vi "Benchmark.vi"() -> ()   [LabVIEW 2023]
uses:
  <vilib>/vision/NI_Vision_Development_Module.lvlib
  WrapperSubVIs/Wrapper.dll
panel:
  out "Time per Image, µs ipp":dbl
  out "Time per Image, µs NI 2 no try catch":dbl
  out "Time per Image, µs 3":dbl
  out "Time per Image, µs 2":dbl
  out "Time per Image, µs original NI":dbl
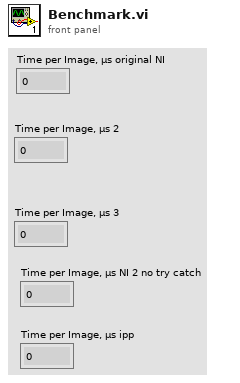
[diagram p1: front panel]
types:
  T1 = typedef "Image Type" = u32
  T2 = typedef "IMAQ Image.ctl" = refnum<image>
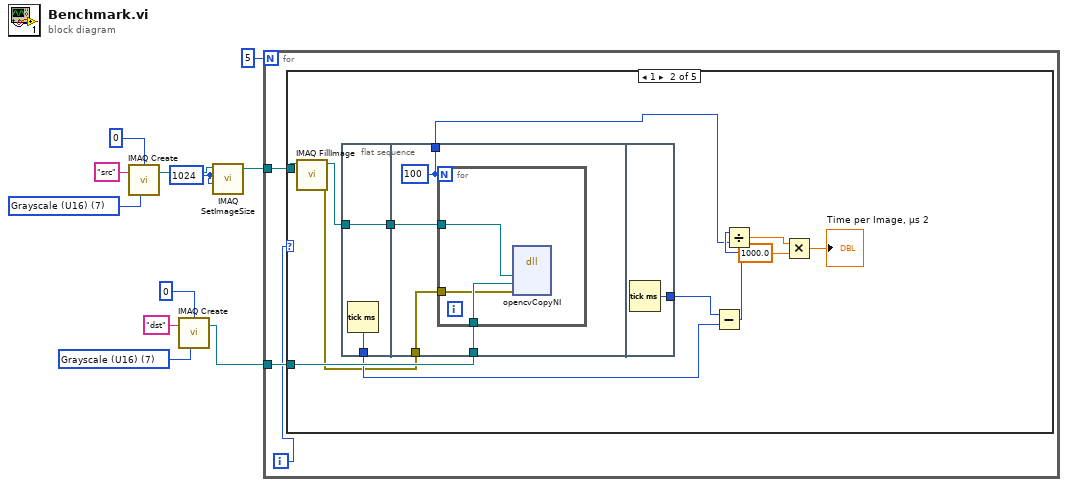
[diagram p0: block diagram]
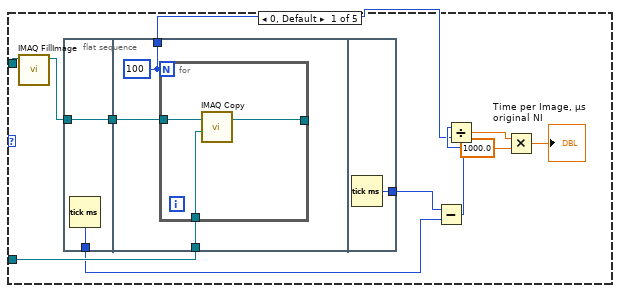
[diagram p2: hidden frame]
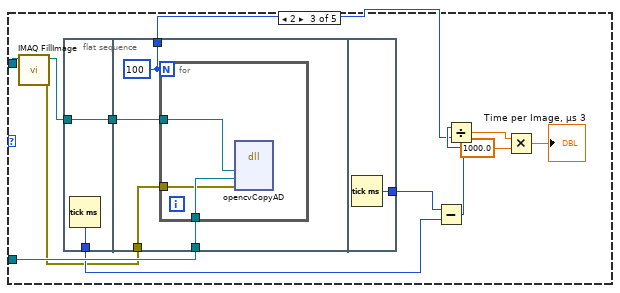
[diagram p3: hidden frame]
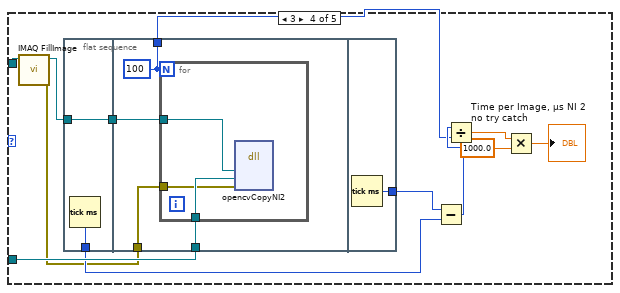
[diagram p4: hidden frame]
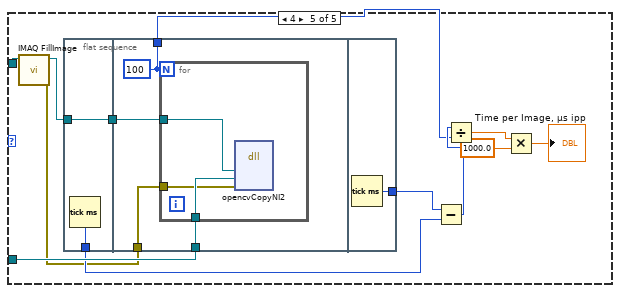
[diagram p5: hidden frame]
diagram:
  w5 = T1 7 items=["Grayscale (U8)", "Grayscale (I16)", "Grayscale (SGL)", "Complex (CSG)", "RGB (U32)", "HSL (U32)", "RGB (U64)", "Grayscale (U16)"] ("Image Type")
  w8 = 1024 ("X Resolution")
  w10 = T1 7 items=["Grayscale (U8)", "Grayscale (I16)", "Grayscale (SGL)", "Complex (CSG)", "RGB (U32)", "HSL (U32)", "RGB (U64)", "Grayscale (U16)"] ("Image Type")
  n1 = call "IMAQ Create"("Border Size"=0, "Image Name"="src", "Image Type"=w10) -> ("New Image"=w9:T2)  [unwired: 2 in, 1 out]
  n2 = call "IMAQ Create"("Border Size"=0, "Image Name"="dst", "Image Type"=w5) -> ("New Image"=w2:T2)  [unwired: 2 in, 1 out]
  n3 = call "IMAQ SetImageSize"("Y Resolution"=w8, "X Resolution"=w8, "Image"=w9) -> ("Image Out"=w3:T2)  [unwired: 2 in, 1 out]
  n4 = for {
    N: 5 -> [_]
    tunnel: w3 -> [w14]
    tunnel: w2 -> [w13]
    i -> [w12]
    n5 = case shown="1" w12 {
      tunnel: w14 -> [w24 w45 w67 w89 w111]
      tunnel: w13 -> [w22 w43 w65 w87 w109]
      frame 0, Default {
        n6 = call "IMAQ FillImage"("Image"=w24) -> ("Image Out"=w23:T2)  [unwired: 9 in, 1 out]
        n7 = flat-sequence {
          tunnel: w23 -> [w27]
          tunnel: [w27] -> w25
          tunnel: [w26] -> w20
          tunnel: w25 -> [w30]
          tunnel: w22 -> [w29]
          tunnel: [w28] -> w18
          tunnel: [w34] -> w21
          frame #0 {
            n8 = Tick Count (ms)() -> (millisecond timer value=w26:u32)
          }
          frame #1 {
            w28 = 100
            n9 = for {
              N: w28 -> [_]
              tunnel: w30 -> [w33]
              tunnel: w29 -> [w32]
              tunnel: [w31] -> _
              n10 = call "IMAQ Copy"("Image Dst"=w32, "Image Src"=w33) -> ("Image Dst Out"=w31:T2)  [unwired: 4 in, 1 out]
            }
          }
          frame #2 {
            n11 = Tick Count (ms)() -> (millisecond timer value=w34:u32)
          }
        }
        n12 = Subtract(x=w21, y=w20) -> (x-y=w19:u32)
        n13 = Divide(x=w19, y=w18) -> (x/y=w17:dbl)
        n14 = Multiply(x=w17, y=1000.0) -> (x*y=→"Time per Image, µs original NI":dbl)
      }
      frame 1 {
        n15 = call "IMAQ FillImage"("Image"=w45) -> ("error out"=w35:errorcluster, "Image Out"=w44:T2)  [unwired: 9 in]
        n16 = flat-sequence {
          tunnel: w44 -> [w48]
          tunnel: [w48] -> w46
          tunnel: [w47] -> w41
          tunnel: w46 -> [w52]
          tunnel: w43 -> [w51]
          tunnel: [w50] -> w39
          tunnel: w35 -> [w49]
          tunnel: [w56] -> w42
          frame #0 {
            n17 = Tick Count (ms)() -> (millisecond timer value=w47:u32)
          }
          frame #1 {
            w50 = 100
            n18 = for {
              N: w50 -> [_]
              tunnel: w52 -> [w55]
              tunnel: w51 -> [w54]
              tunnel: w49 -> [w53]
              n19 = dll-call lib="C:/Users/Andrey/Desktop/xe2/WrapperSubVIs/Wrapper.dll" fn="opencvCopyNI"("src"=w55, "dst"=w54, "err"=w53) -> ()  [unwired: 7 in, 2 out]
            }
          }
          frame #2 {
            n20 = Tick Count (ms)() -> (millisecond timer value=w56:u32)
          }
        }
        n21 = Subtract(x=w42, y=w41) -> (x-y=w40:u32)
        n22 = Divide(x=w40, y=w39) -> (x/y=w38:dbl)
        n23 = Multiply(x=w38, y=1000.0) -> (x*y=→"Time per Image, µs 2":dbl)
      }
      frame 2 {
        n24 = call "IMAQ FillImage"("Image"=w67) -> ("error out"=w57:errorcluster, "Image Out"=w66:T2)  [unwired: 9 in]
        n25 = flat-sequence {
          tunnel: w66 -> [w70]
          tunnel: [w70] -> w68
          tunnel: [w69] -> w63
          tunnel: w68 -> [w74]
          tunnel: w65 -> [w73]
          tunnel: [w72] -> w61
          tunnel: w57 -> [w71]
          tunnel: [w78] -> w64
          frame #0 {
            n26 = Tick Count (ms)() -> (millisecond timer value=w69:u32)
          }
          frame #1 {
            w72 = 100
            n27 = for {
              N: w72 -> [_]
              tunnel: w74 -> [w77]
              tunnel: w73 -> [w76]
              tunnel: w71 -> [w75]
              n28 = dll-call lib="C:/Users/Andrey/Desktop/xe2/WrapperSubVIs/Wrapper.dll" fn="opencvCopyAD"("src"=w77, "dst"=w76, "err"=w75) -> ()  [unwired: 7 in, 2 out]
            }
          }
          frame #2 {
            n29 = Tick Count (ms)() -> (millisecond timer value=w78:u32)
          }
        }
        n30 = Subtract(x=w64, y=w63) -> (x-y=w62:u32)
        n31 = Divide(x=w62, y=w61) -> (x/y=w60:dbl)
        n32 = Multiply(x=w60, y=1000.0) -> (x*y=→"Time per Image, µs 3":dbl)
      }
      frame 3 {
        n33 = call "IMAQ FillImage"("Image"=w89) -> ("error out"=w79:errorcluster, "Image Out"=w88:T2)  [unwired: 9 in]
        n34 = flat-sequence {
          tunnel: w88 -> [w92]
          tunnel: [w92] -> w90
          tunnel: [w91] -> w85
          tunnel: w90 -> [w96]
          tunnel: w87 -> [w95]
          tunnel: [w94] -> w83
          tunnel: w79 -> [w93]
          tunnel: [w100] -> w86
          frame #0 {
            n35 = Tick Count (ms)() -> (millisecond timer value=w91:u32)
          }
          frame #1 {
            w94 = 100
            n36 = for {
              N: w94 -> [_]
              tunnel: w96 -> [w99]
              tunnel: w95 -> [w98]
              tunnel: w93 -> [w97]
              n37 = dll-call lib="C:/Users/Andrey/Desktop/xe2/WrapperSubVIs/Wrapper.dll" fn="opencvCopyNI2"("src"=w99, "dst"=w98, "err"=w97) -> ()  [unwired: 7 in, 2 out]
            }
          }
          frame #2 {
            n38 = Tick Count (ms)() -> (millisecond timer value=w100:u32)
          }
        }
        n39 = Subtract(x=w86, y=w85) -> (x-y=w84:u32)
        n40 = Divide(x=w84, y=w83) -> (x/y=w82:dbl)
        n41 = Multiply(x=w82, y=1000.0) -> (x*y=→"Time per Image, µs NI 2 no try catch":dbl)
      }
      frame 4 {
        n42 = call "IMAQ FillImage"("Image"=w111) -> ("error out"=w101:errorcluster, "Image Out"=w110:T2)  [unwired: 9 in]
        n43 = flat-sequence {
          tunnel: w110 -> [w114]
          tunnel: [w114] -> w112
          tunnel: [w113] -> w107
          tunnel: w112 -> [w118]
          tunnel: w109 -> [w117]
          tunnel: [w116] -> w105
          tunnel: w101 -> [w115]
          tunnel: [w122] -> w108
          frame #0 {
            n44 = Tick Count (ms)() -> (millisecond timer value=w113:u32)
          }
          frame #1 {
            w116 = 100
            n45 = for {
              N: w116 -> [_]
              tunnel: w118 -> [w121]
              tunnel: w117 -> [w120]
              tunnel: w115 -> [w119]
              n46 = dll-call lib="C:/Users/Andrey/Desktop/xe2/WrapperSubVIs/Wrapper.dll" fn="opencvCopyNI2"("src"=w121, "dst"=w120, "err"=w119) -> ()  [unwired: 7 in, 2 out]
            }
          }
          frame #2 {
            n47 = Tick Count (ms)() -> (millisecond timer value=w122:u32)
          }
        }
        n48 = Subtract(x=w108, y=w107) -> (x-y=w106:u32)
        n49 = Divide(x=w106, y=w105) -> (x/y=w104:dbl)
        n50 = Multiply(x=w104, y=1000.0) -> (x*y=→"Time per Image, µs ipp":dbl)
      }
    }
  }
